vi "XLP80_Action_EnableCVMTestmode_B.vi"(7 "but_Enable reading cell voltage":bool caption="Enable reading cell voltage", 8 "err in":errorcluster) -> (0 "err out":errorcluster)   [LabVIEW 2021]
uses:
  XLP80_FGlob/1886_FGlob_TDefs_Enum_FGlobItems.ctl
  XLP80_FGlob/1886_FGlob_TDefEnumCANWriteItems.ctl
  XLP80_State_V001.llb/XLP80_State_Globals.vi
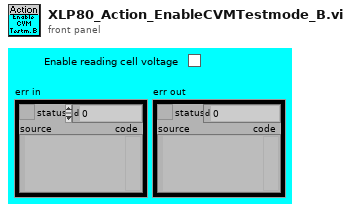
[diagram p1: front panel]
types:
  T1 = typedef "1886_FGlob_TDefs_Enum_FGlobItems.ctl" = enum16{"Put one", "Put all", "Recall one", "Recall all"}
  T2 = typedef "1886_FGlob_TDefEnumCANWriteItems.ctl" = enum16{"LV_Testmode_Select", "LV_A_71_Current_Out_Set", "LV_A_71_Voltage_In_Set", "LV_A_71_Voltage_Out_Set", "LV_H_51_STK_CellVoltages_Enable", "S80_BP_s_Taster_Start_Status"}
  T3 = typedef "XLP80_State_TDefEnumGlobalState.ctl" = enum16{"HV & Software", "Basis Funktion", "Power Management", "Operational Mode", "Shutdown", "Alarm"}
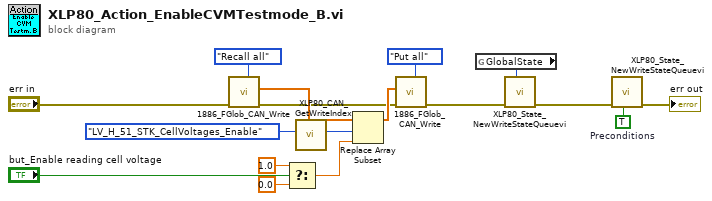
[diagram p0: block diagram]
diagram:
  w3 = TRUE  # Preconditions
  n1 = call "1886_FGlob_CAN_Write.vi"("Function (Recall One)"=1886_FGlob_TDefs_Enum_FGlobItems."Recall all", "err in"="err in") -> ("err out"=w11:errorcluster, "AO Values OUT"=w13:dbl[])  [unwired: 7 in, 1 out]
  n2 = Select(t=1.0 ("new element/subarray"), s="but_Enable reading cell voltage", f=0.0 ("new element/subarray")) -> (s? t:f=w6:dbl)
  n3 = call "XLP80_CAN_GetWriteIndex.vi"("CAN Write Items"=1886_FGlob_TDefEnumCANWriteItems."LV_H_51_STK_CellVoltages_Enable" ("CAN Write Items Testmode_A")) -> ("Index"=w16:i32)  [unwired: 10 in]
  n4 = Replace Array Subset(array=w13, new element=w6, index=w16) -> (w12:dbl[])
  n5 = call "1886_FGlob_CAN_Write.vi"("Function (Recall One)"=1886_FGlob_TDefs_Enum_FGlobItems."Put all", "err in"=w11, "AO Values IN"=w12) -> ("err out"=w1:errorcluster)  [unwired: 6 in, 2 out]
  n6 = global read "XLP80_State_Globals.vi" "GlobalState"() -> (w5:T3)
  n7 = call "XLP80_State_NewWriteStateQueuevi.vi"("GlobalState"=w5, "err in"=w1) -> ("err out"=w4:errorcluster)  [unwired: 9 in]
  n8 = call "XLP80_State_NewWriteStateQueuevi.vi"("Preconditions"=w3, "err in"=w4) -> ("err out"=→"err out":errorcluster)  [unwired: 9 in]
